vi "UnlinkNode.vi"(8 "error in":errorcluster, 10 "child in":T1, 11 "parent in":T1) -> (0 "error out":errorcluster, 2 "child out":T1, 3 "parent out":T1)   [LabVIEW 2023, in "CEF.lvlib" / "CEF_Node.lvclass"]
doc: "Breaks the link between a child and a parent node. Removing the reference to each other in both nodes.Copyright 2017 National Instruments Corporation\n\nLicensed under the Apache License, Version 2.0 (the \"License\"); you may not use this file except in compliance with the License. You may obtain a copy of the License at http://www.apache.org/licenses/LICENSE-2.0\nUnless required by applicable law or agreed to in writing, software distributed under the License is distributed on an \"AS IS\" BASIS, WITHOUT WARRANTIES OR CONDITIONS OF ANY KIND, either express or implied. See the License for the specific language governing permissions and limitations under the License."
uses:
  CEF_Node.lvclass
  NodeRef.ctl
  CEF_Node.lvclass/CEF_Node.ctl
  ReadChildren.vi
  WriteParent.vi
  WriteChildren.vi
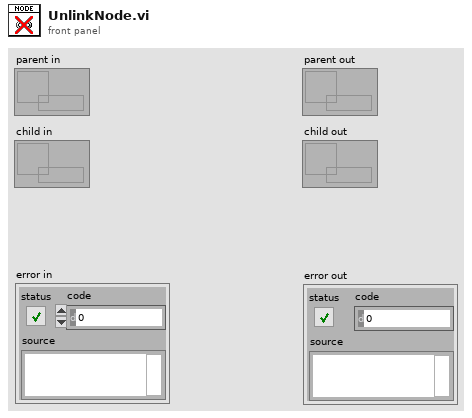
[diagram p1: front panel]
types:
  T1 = typedef "CEF.lvlib/CEF_Node.lvclass/NodeRef.ctl" = refnum<data-value>
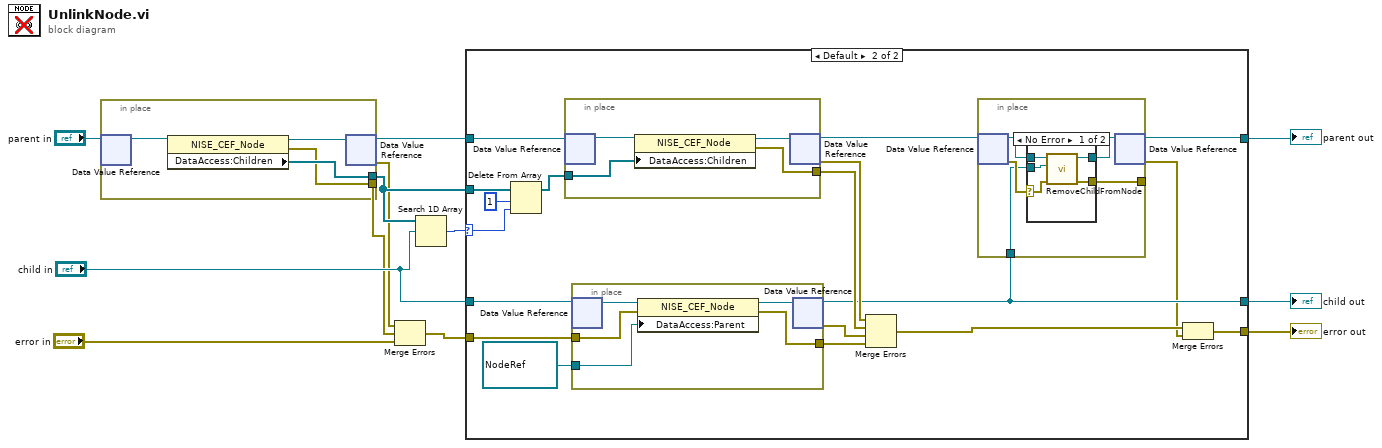
[diagram p0: block diagram]
diagram:
  n1 = in-place {
    in-place-border: [w14] -> w10
    in-place-border: [w13] -> w2
    n2 = in-place-dvr #1("parent in") -> (w16:refnum<class "CEF_Node.lvclass">)  [unwired: 1 out]
    n3 = property class="NISE_CEF_Node"(reference=w16) -> (reference out=w15:refnum<class "CEF_Node.lvclass">, error out=w13:errorcluster, "DataAccess:Children"=w14:T1[])  [unwired: 1 in]
    n4 = in-place-dvr #1(w15) -> (w11:T1, w1:errorcluster)
  }
  n5 = Merge Errors(w1, w2, "error in") -> (w3:errorcluster)
  n6 = Search 1D Array(1D array=w10, element="child in") -> (index of element=w12:i32)  [unwired: 1 in]
  n7 = case shown="Default" w12 {
    selector: w12 -> [_ w33]
    tunnel: "child in" -> [w17 w37]
    tunnel: w3 -> [w19 w36]
    tunnel: [w19 w23] -> w9
    tunnel: w11 -> [w18 w31]
    tunnel: [w18 w25] -> w5
    tunnel: [w17 w24] -> w6
    tunnel: w10 -> [_ w35]
    frame -1 {
    }
    frame Default {
      n8 = Delete From Array(array=w35, length=1, index=w33) -> (array with subset deleted=w32:T1[])  [unwired: 1 out]
      n9 = in-place {
        in-place-border: w32 -> [w51]
        in-place-border: [w50] -> w30
        n10 = in-place-dvr #2(w31) -> (w53:refnum<class "CEF_Node.lvclass">)  [unwired: 1 out]
        n11 = property class="NISE_CEF_Node"(reference=w53, "DataAccess:Children"=w51) -> (reference out=w52:refnum<class "CEF_Node.lvclass">, error out=w50:errorcluster)  [unwired: 1 in]
        n12 = in-place-dvr #2(w52) -> (w26:T1, w29:errorcluster)
      }
      n13 = in-place {
        in-place-border: w36 -> [w57]
        in-place-border: [w55] -> w28
        in-place-border: T1 refnum ("Parent") -> [w54]
        n14 = in-place-dvr #3(w37) -> (w58:refnum<class "CEF_Node.lvclass">)  [unwired: 1 out]
        n15 = property class="NISE_CEF_Node"(reference=w58, error in=w57, "DataAccess:Parent"=w54) -> (reference out=w56:refnum<class "CEF_Node.lvclass">, error out=w55:errorcluster)
        n16 = in-place-dvr #3(w56) -> (w24:T1, w27:errorcluster)
      }
      n17 = Merge Errors(w29, w30, w27, w28) -> (w22:errorcluster)
      n18 = in-place {
        in-place-border: [w42] -> _
        in-place-border: w24 -> [w38]
        n19 = in-place-dvr #4(w26) -> (w41:refnum<class "CEF_Node.lvclass">, w39:errorcluster)
        n20 = case shown="No Error" w39 {
          selector: w39 -> [w43 w48]
          tunnel: [w47 w48] -> w42
          tunnel: w41 -> [w46 w49]
          tunnel: [w45 w49] -> w40
          tunnel: w38 -> [w44 _]
          frame No Error {
            n21 = call-dynamic "RemoveChildFromNode.vi"("error in"=w43, "removed child"=w44, "CEF_Node in"=w46) -> ("error out"=w47:errorcluster, "CEF_Node out"=w45:refnum<class "CEF_Node.lvclass">)  [unwired: 7 in]
          }
          frame Error {
          }
        }
        n22 = in-place-dvr #4(w40) -> (w25:T1, w21:errorcluster)
      }
      n23 = Merge Errors(w22, w21) -> (w23:errorcluster)
    }
  }
  "child out" <- w6
  "parent out" <- w5
  "error out" <- w9
